vi "Calib_General_Setup.vi"(0 "Reference instrument":T3={"high limit (10V)"=4.0, "low limit (-10V)"=0.0, "Ch No"=4, "Off ch no"=0, "Calib filename"=path "", "Ref Instrument type"=enum."Enter Value"} {"Off ch no" min=0 max=1; "Ch No" min=0 max=7; "low limit (-10V)" min=-10 max=10 format="%.3f"; "high limit (10V)" min=-10 max=10 format="%.3f"}, 1 "Requested No of samples":i32=128 min=0 step=1, 2 "Sampling rate (Hz)":sgl=1000.0 format="%.2f", 5 "2nd ref instrument":T2={"2nd Ref type"=enum."LDA", "2nd inst present"=TRUE}, 9 "Temp":dbl=20.0 format="%.1f", 11 "Board type":T4=enum."Local ADAM", 12 "Abs Press (mbar)":dbl=1005.0 format="%.2f") -> (8 "Output string":string, 10 "LDA Data":bool)   [LabVIEW 2010]
uses:
  Controls/Board_Types.ctl
  Controls/Ref_Inst_type.ctl
  Controls/Graph_Type.ctl
  Globals/Meas_global.vi
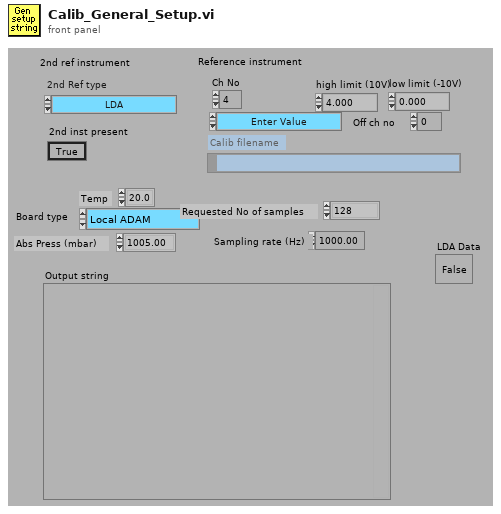
[diagram p1: front panel]
types:
  T1 = typedef "Ref_Inst_type.ctl" = enum16{"Propellor anemometer", "Pressure Transducer", "Raw voltage", "Pitot-static tube", "Preston tube", "Generic Linear", "Generic Polynomial", "Thermocouple", "LDA", "Enter Value", "ADAM Channel"}
  T2 = cluster{"2nd Ref type":T1, "2nd inst present":bool}
  T3 = cluster{"high limit (10V)":sgl, "low limit (-10V)":sgl, "Ch No":i16, "Off ch no":i8, "Calib filename":path, "Ref Instrument type":T1}
  T4 = typedef "Board_Types.ctl" = enum16{"Simulate", "Local ADAM", "Server ADAM", "NI-DAQmx", "NI-DAQmxBase", "ADC488", "DT LV-link"}
  T5 = typedef "Graph_Type.ctl" = enum16{"Show no graph", "Voltage trace", "Velocity trace", "Vel histogram", "Spectrum", "f.E(f) v Log f", "Auto-Corr"}
  T6 = cluster{"Plot 1":u16, "Plot 2":u16, "Save graph":u16, "Plot Type":T5}
  T7 = enum16{"From String to Cluster", "From Cluster to String"}
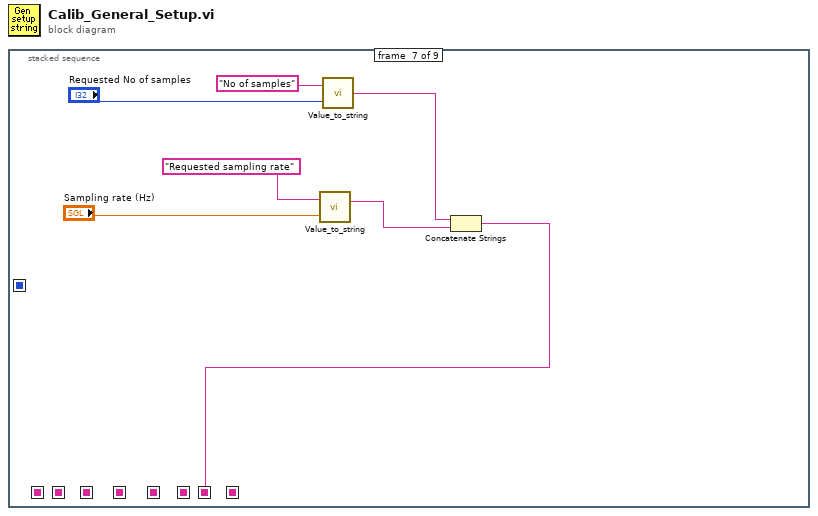
[diagram p0: block diagram]
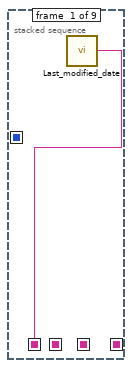
[diagram p2: hidden frame]
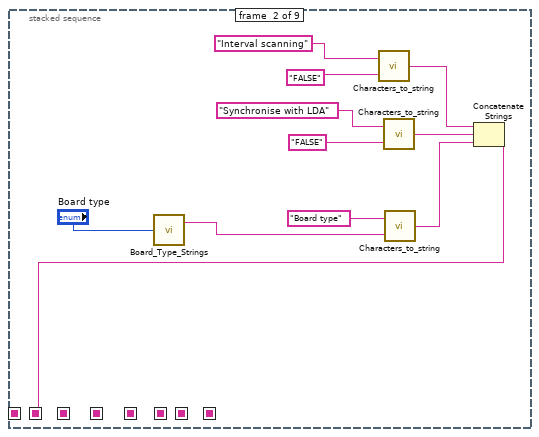
[diagram p3: hidden frame]
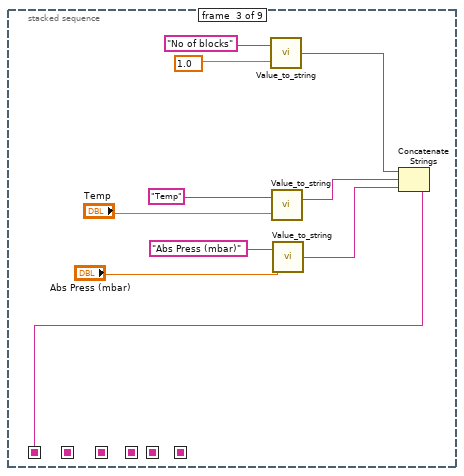
[diagram p4: hidden frame]
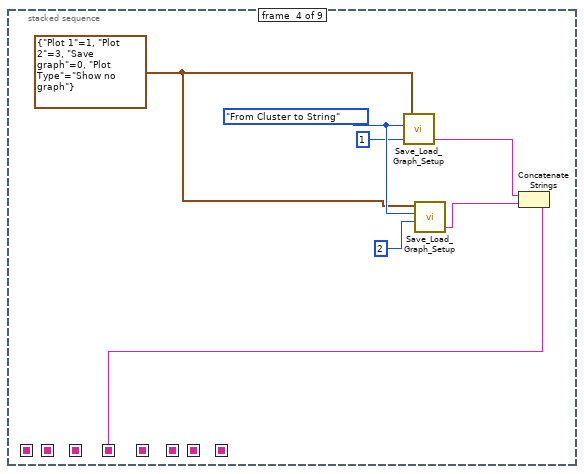
[diagram p5: hidden frame]
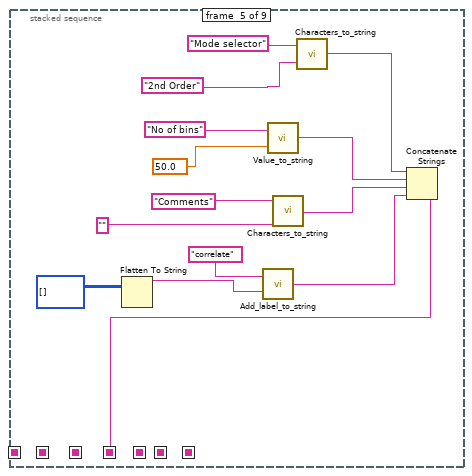
[diagram p6: hidden frame]
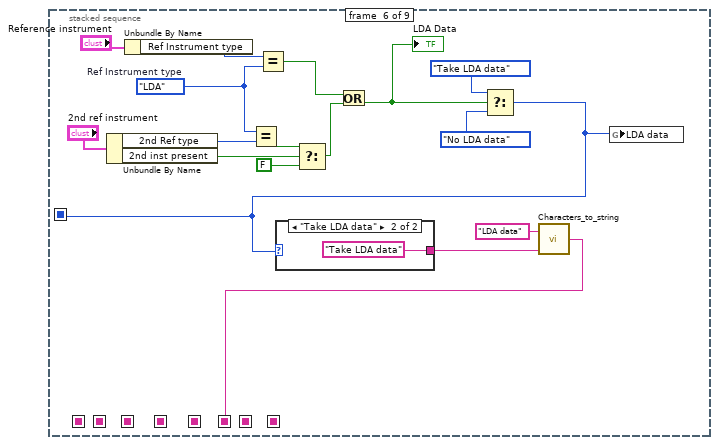
[diagram p7: hidden frame]
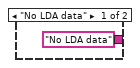
[diagram p8: hidden frame]
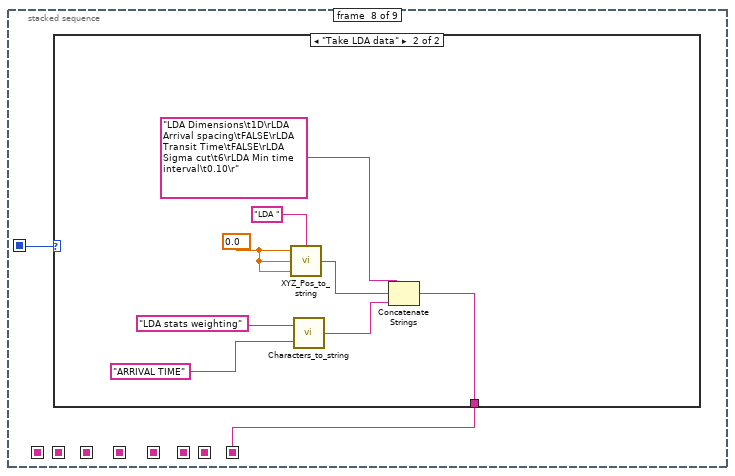
[diagram p9: hidden frame]
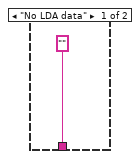
[diagram p10: hidden frame]
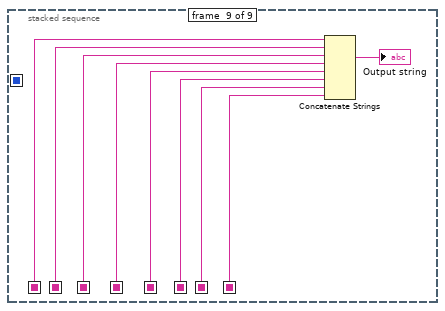
[diagram p11: hidden frame]
diagram:
  n1 = stacked-sequence {
    seq-local: [_ _ w21 _ _ _ _ _ _] -> [_ _ _ _ _ _ _ _ w89]
    seq-local: [_ w6 _ _ _ _ _ _ _] -> [_ _ _ _ _ _ _ _ w88]
    seq-local: [_ _ _ _ _ w58 _ _ _] -> [_ _ _ _ _ _ _ _ w84]
    seq-local: [_ _ _ _ _ _ w68 _ _] -> [_ _ _ _ _ _ _ _ w83]
    seq-local: [_ _ _ w24 _ _ _ _ _] -> [_ _ _ _ _ _ _ _ w86]
    seq-local: [_ _ _ _ w34 _ _ _ _] -> [_ _ _ _ _ _ _ _ w85]
    seq-local: [w1 _ _ _ _ _ _ _ _] -> [_ _ _ _ _ _ _ _ w82]
    seq-local: [_ _ _ _ _ w45 _ _ _] -> [_ _ _ _ _ _ _ w71 _]
    seq-local: [_ _ _ _ _ _ _ w70 _] -> [_ _ _ _ _ _ _ _ w81]
    frame #0 {
      n2 = call "Last_modified_date.vi"() -> ("Output string"=w1:string)  [unwired: 1 in, 1 out]
    }
    frame #1 {
      n3 = call "Board_Type_Strings.vi"("Board type"="Board type") -> ("Board String"=w2:string)  [unwired: 1 out]
      n4 = call "Characters_to_string.vi"("Characters to write"="FALSE", "Label for characters"="Interval scanning") -> ("Output string"=w9:string)
      n5 = call "Characters_to_string.vi"("Characters to write"="FALSE", "Label for characters"="Synchronise with LDA") -> ("Output string"=w8:string)
      n6 = call "Characters_to_string.vi"("Characters to write"=w2, "Label for characters"="Board type") -> ("Output string"=w7:string)
      n7 = Concatenate Strings(w9, w8, w7) -> (w6:string)
    }
    frame #2 {
      n8 = call "Value_to_string.vi"("Value"=1.0, "Label for value"="No of blocks") -> ("Output string"=w15:string)  [unwired: 1 in]
      n9 = call "Value_to_string.vi"("Value"="Temp", "Label for value"="Temp") -> ("Output string"=w18:string)  [unwired: 1 in]
      n10 = call "Value_to_string.vi"("Value"="Abs Press (mbar)", "Label for value"="Abs Press (mbar)") -> ("Output string"=w17:string)  [unwired: 1 in]
      n11 = Concatenate Strings(w15, w18, w17) -> (w21:string)
    }
    frame #3 {
      w23 = T6 {"Plot 1"=1, "Plot 2"=3, "Save graph"=0, "Plot Type"=enum."Show no graph"} ("Graph in")
      w27 = T7."From Cluster to String" ("Mode")
      n12 = call "Save_Load_Graph_Setup.vi"("Graph Number"=1, "Mode"=w27, "Graph in"=w23) -> ("Setup String Out"=w29:string)  [unwired: 1 in, 2 out]
      n13 = call "Save_Load_Graph_Setup.vi"("Graph Number"=2, "Mode"=w27, "Graph in"=w23) -> ("Setup String Out"=w28:string)  [unwired: 1 in, 2 out]
      n14 = Concatenate Strings(w29, w28) -> (w24:string)
    }
    frame #4 {
      n15 = Flatten To String(anything=i8[][] [] ("correlate")) -> (data string=w30:string)  [unwired: 1 in, 4 out]
      n16 = call "Add_label_to_string.vi"("String to write"=w30, "File Label"="correlate") -> ("Output string"=w35:string)
      n17 = call "Value_to_string.vi"("Value"=50.0 ("Bins"), "Label for value"="No of bins") -> ("Output string"=w42:string)  [unwired: 1 in]
      n18 = call "Characters_to_string.vi"("Characters to write"="" ("Comments"), "Label for characters"="Comments") -> ("Output string"=w37:string)
      n19 = call "Characters_to_string.vi"("Characters to write"="2nd Order", "Label for characters"="Mode selector") -> ("Output string"=w39:string)
      n20 = Concatenate Strings(w39, w42, w37, w35) -> (w34:string)
    }
    frame #5 {
      w44 = Ref_Inst_type."LDA"  # Ref Instrument type
      n21 = Unbundle By Name("2nd ref instrument") -> ("2nd Ref type"=w53:T1, "2nd inst present"=w54:bool)
      n22 = Unbundle By Name("Reference instrument") -> ("Ref Instrument type"=w55:T1)
      n23 = Equal?(x=w44, y=w53) -> (x = y?=w52:bool)
      n24 = Equal?(x=w55, y=w44) -> (x = y?=w49:bool)
      n25 = Select(t=w52, s=w54, f=FALSE) -> (s? t:f=w50:bool)
      n26 = Or(x=w49, y=w50) -> (x .or. y?=w46:bool)
      "LDA Data" <- w46
      n27 = Select(t=enum16{"No LDA data", "Take LDA data"}."Take LDA data" ("LDA data"), s=w46, f=enum16{"No LDA data", "Take LDA data"}."No LDA data" ("LDA data")) -> (s? t:f=w45:enum16{"No LDA data", "Take LDA data"})
      n28 = case shown="\"Take LDA data\"" w45 {
        tunnel: ["No LDA data" "Take LDA data"] -> w59
        frame "No LDA data" {
        }
        frame "Take LDA data" {
        }
      }
      n29 = call "Characters_to_string.vi"("Characters to write"=w59, "Label for characters"="LDA data") -> ("Output string"=w58:string)
      n30 = global write "Meas_global.vi" "LDA data"(w45) -> ()
    }
    frame #6 {
      n31 = call "Value_to_string.vi"("Value"="Sampling rate (Hz)", "Label for value"="Requested sampling rate") -> ("Output string"=w66:string)  [unwired: 1 in]
      n32 = call "Value_to_string.vi"("Value"="Requested No of samples", "Label for value"="No of samples") -> ("Output string"=w67:string)  [unwired: 1 in]
      n33 = Concatenate Strings(w67, w66) -> (w68:string)
    }
    frame #7 {
      n34 = case shown="\"Take LDA data\"" w71 {
        tunnel: ["" w74] -> w70
        frame "No LDA data" {
        }
        frame "Take LDA data" {
          w80 = 0.0 ("X")
          n35 = call "XYZ_Pos_to_string.vi"("Position label"="LDA ", "Z"=w80, "Y"=w80, "X"=w80) -> ("Output string"=w76:string)
          n36 = call "Characters_to_string.vi"("Characters to write"="ARRIVAL TIME" ("LDA stats type"), "Label for characters"="LDA stats weighting") -> ("Output string"=w75:string)
          n37 = Concatenate Strings("LDA Dimensions\t1D\rLDA Arrival spacing\tFALSE\rLDA Transit Time\tFALSE\rLDA Sigma cut\t6\rLDA Min time interval\t0.10\r" ("String"), w76, w75) -> (w74:string)
        }
      }
    }
    frame #8 {
      n38 = Concatenate Strings(w82, w88, w89, w86, w85, w84, w83, w81) -> (→"Output string":string)
    }
  }
